vi "Build FIU Section.vi"(6 "Cancelled?":bool, 8 "error in (no error)":errorcluster, 9 "Card Position in":T1 {"Slot #" max=15}, 10 "Name in":string, 11 "Node Ptr in":u64) -> (0 "error out":errorcluster)   [LabVIEW 2014, in "SLSC configuration System Explorer.lvlib"]
uses:
  SLSC configuration System Explorer.lvlib
  Type Defs/Card Position.ctl
  Shared/SPI Utility/Slot #.ctl
  <vilib>/NI Veristand/Custom Device API/Custom Device Channel.ctl
  <vilib>/NI Veristand/Custom Device API/Custom Device Channel Type.ctl
  Shared/Constants.vi
  <vilib>/NI Veristand/Custom Device API/Set Item Property (U16).vi
  <vilib>/NI Veristand/Custom Device API/Custom Device API.lvlib
  Shared/SLSC configuration Shared.lvlib
  <vilib>/NI Veristand/Custom Device Tools/Custom Device Utility Library/Custom Device Utility Library.lvlib
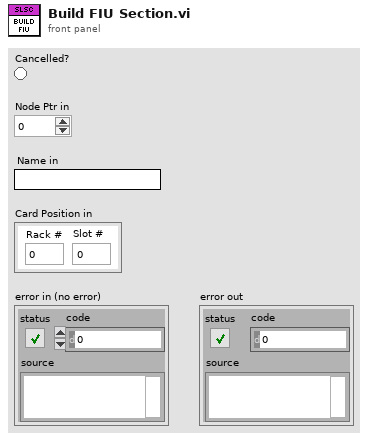
[diagram p1: front panel]
types:
  T1 = typedef "SLSC configuration Shared.lvlib/Card Position.ctl" = cluster{"Rack #":u8, "Slot #":T2}
  T2 = typedef "SLSC configuration Shared.lvlib/Slot #.ctl" = u8
  T3 = typedef "Custom Device API.lvlib/Custom Device Channel Type.ctl" = enum16{"Input", "Output"}
  T4 = typedef "Custom Device API.lvlib/Custom Device Channel.ctl" = cluster{"Type":T3, "Units":string, "Default Value":dbl, "Faultable":bool, "Scalable":bool}
  T5 = typedef "Custom Device API.lvlib/Custom Device Item Ref.ctl" = u64
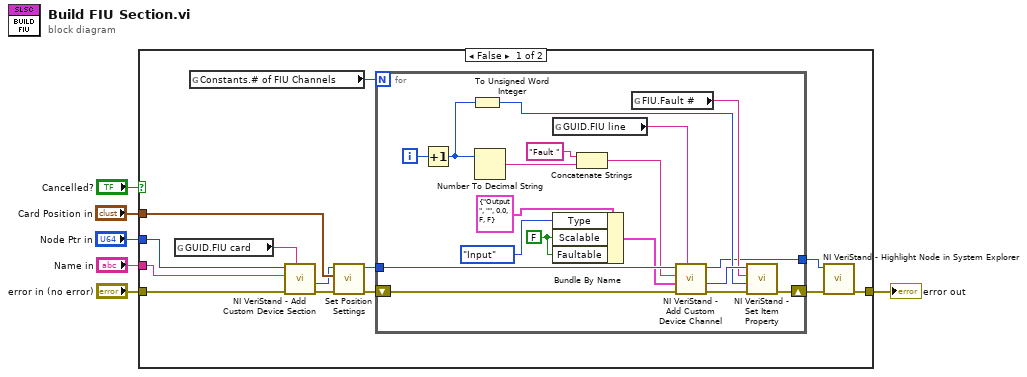
[diagram p0: block diagram]
diagram:
  n1 = case shown="False" "Cancelled?" {
    tunnel: "Node Ptr in" -> [w19 _]
    tunnel: "Name in" -> [w18 _]
    tunnel: "error in (no error)" -> [w17 w38]
    tunnel: "Card Position in" -> [w8 _]
    tunnel: [w13 w38] -> w5
    frame False {
      n2 = global read "Constants.vi" "GUID.FIU card"() -> (w16:string)
      n3 = global read "Constants.vi" "Constants.# of FIU Channels"() -> (w12:u8)
      n4 = call <vilib>:"NI VeriStand - Add Custom Device Section.vi"("GUID (Default Section)"=w16, "error in (no error)"=w17, "Section Name"=w18, "Parent Ref in"=w19) -> ("error out"=w11:errorcluster, "Section Ptr"=w7:T5)  [unwired: 4 in, 2 out]
      n5 = call "Set Position Settings.vi"("error in (no error)"=w11, "Card Position"=w8, "Item Ref in"=w7) -> ("error out"=w9:errorcluster, "Item Ref out"=w10:T5)  [unwired: 7 in]
      n6 = for {
        N: w12 -> [_]
        shift-right: [w29] -> w15
        shift-left: w9 -> [w35]
        tunnel: w10 -> [w36]
        tunnel: [w20] -> w14
        i -> [w37]
        w21 = FALSE ("Scalable")
        n7 = Increment(x=w37) -> (x+1=w26:i32)
        n8 = To Unsigned Word Integer(number=w26) -> (unsigned 16bit integer=w25:u16)
        n9 = Number To Decimal String(number=w26) -> (decimal integer string=w33:string)  [unwired: 1 in]
        n10 = global read "Constants.vi" "GUID.FIU line"() -> (w34:string)
        n11 = Bundle By Name(cluster=T4 {"Type"=enum."Output", "Units"="", "Default Value"=0.0, "Faultable"=FALSE, "Scalable"=FALSE} ("Channel"), "Type"=Custom_Device_Channel_Type."Input", "Scalable"=w21, "Faultable"=w21) -> (w23:T4)
        n12 = Concatenate Strings("Fault " ("Channel Name"), w33) -> (w31:string)
        n13 = global read "Constants.vi" "FIU.Fault #"() -> (w27:string)
        n14 = call <vilib>:"NI VeriStand - Add Custom Device Channel.vi"("GUID (Default Channel)"=w34, "error in (no error)"=w35, "Channel"=w23, "Channel Name"=w31, "Parent Ref in"=w36) -> ("error out"=w30:errorcluster, "Channel Ref"=w28:T5, "Parent Ref out"=w20:T5)  [unwired: 3 in, 1 out]
        n15 = call-poly <vilib>:"NI VeriStand - Set Item Property.vi"("error in (no error)"=w30, "Value"=w25, "Property Name"=w27, "Item Ref in"=w28) -> ("error out"=w29:errorcluster)  [unwired: 5 in, 2 out]
      }
      n16 = call <vilib>:"NI VeriStand - Highlight Node in System Explorer.vi"("error in (no error)"=w15, "Item Ref in"=w14) -> ("error out"=w13:errorcluster)  [unwired: 8 in, 1 out]
    }
    frame True {
    }
  }
  "error out" <- w5
